vi "newinit.vi"(10 "error in":errorcluster, 11 "Automation Refnum":refnum<k7>) -> (1 "error out":errorcluster, 2 "Detected?":bool, 3 "xphyspecLib.IXPhySpec out":refnum<k7>)   [LabVIEW 2019]
panel:
  out "Error message":string
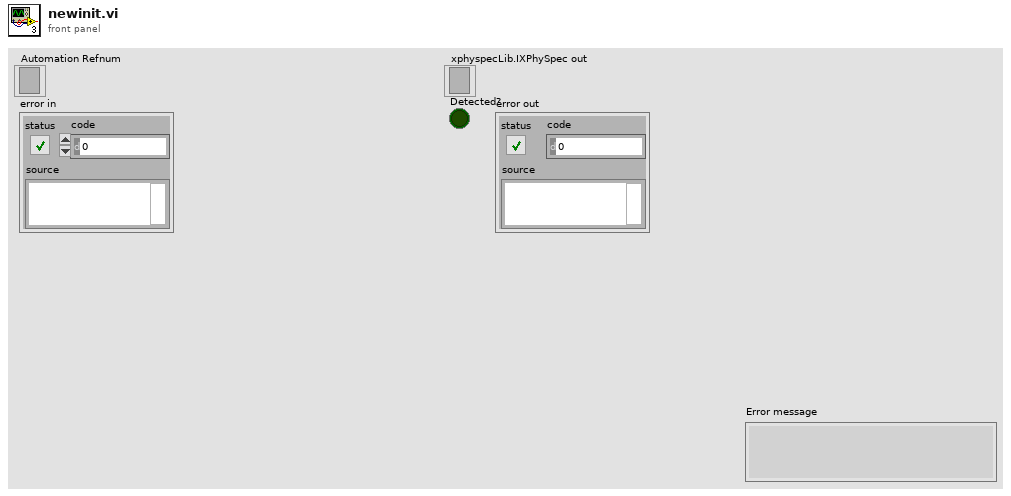
[diagram p1: front panel]
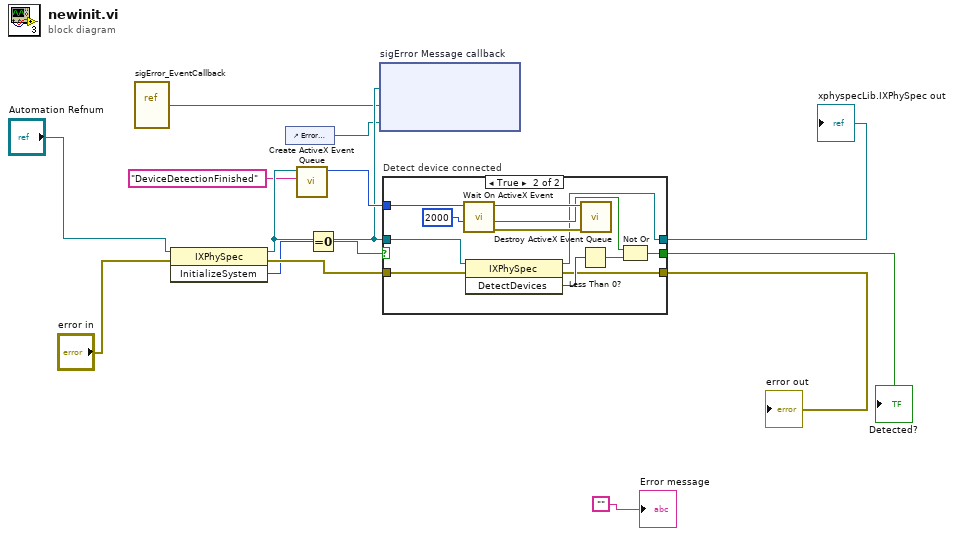
[diagram p0: block diagram]
diagram:
  n1 = vi-ref "sigError_EventCallback.vi"() -> ("vi reference"=w6:refnum<vi>)
  n2 = invoke class="IXPhySpec" method="InitializeSystem"(reference="Automation Refnum", error in="error in") -> (reference out=w9:refnum<k7>, error out=w10:errorcluster, "InitializeSystem"=w4:i32)  [unwired: 1 in]
  n3 = control-ref of="Error message"() -> (w5:refnum<vi>)
  n4 = call <vilib>:"Create ActiveX Event Queue.vi"("Event Name"="DeviceDetectionFinished", "Automation Refnum"=w9) -> ("Event Queue"=w11:i32)  [unwired: 4 in, 1 out]
  n5 = Equal To 0?(x=w4) -> (x = 0?=w8:bool)
  n6 = node "sigError Message callback"(w9, w6, w5) -> ()  [unwired: 2 in, 2 out]
  n7 = case "Detect device connected" shown="True" w8 {
    selector: w8 -> [w17 _]
    tunnel: w9 -> [w16 w29]
    tunnel: w10 -> [w15 w28]
    tunnel: w11 -> [_ w25]
    tunnel: [w16 w20] -> w12
    tunnel: [w15 w19] -> w13
    tunnel: [w17 w18] -> w14
    frame False {
    }
    frame True {
      n8 = call <vilib>:"Wait On ActiveX Event.vi"("ms Timeout (-1)"=2000, "Event Queue"=w25) -> ("error out"=w24:errorcluster, "Timed Out"=w22:bool, "Event Queue Out"=w26:i32)  [unwired: 2 in, 1 out]
      n9 = invoke class="IXPhySpec" method="DetectDevices"(reference=w29, error in=w28) -> (reference out=w20:refnum<k7>, error out=w19:errorcluster, "DetectDevices"=w23:i32)  [unwired: 1 in]
      n10 = Less Than 0?(x=w23) -> (x < 0?=w21:bool)
      n11 = call <vilib>:"Destroy ActiveX Event Queue.vi"("error in (no error)"=w24, "Event Queue"=w26) -> ()  [unwired: 5 in, 1 out]
      n12 = Not Or(1:w21, 2:w22) -> (0:w18:bool)
    }
  }
  "xphyspecLib.IXPhySpec out" <- w12
  "Detected?" <- w14
  "error out" <- w13
  "Error message" <- ""
